vi "convert_image_to_U16.vi"(7 "File Path":path, 8 "error in (no error)":errorcluster, 9 "Image Name":string="untitled", 10 "Convert to U16?":bool, 11 "Image":T1) -> (0 "error out":errorcluster, 2 "unsigned 16bit integer":u16[][](array[numeric]), 3 "Image Out":T1)   [LabVIEW 2013, in "Hamamatsu_C9100-13.lvclass"]
uses:
  Hamamatsu_C9100-13/Hamamatsu_C9100-13.lvclass
  <vilib>/vision/Image Controls.llb/IMAQ Image.ctl
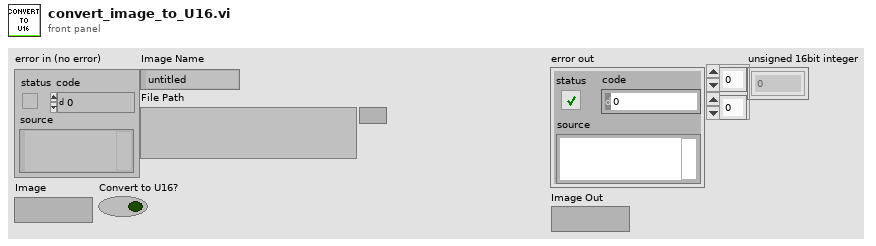
[diagram p1: front panel]
types:
  T1 = typedef "IMAQ Image.ctl" = refnum<image>
  T2 = typedef "Image Type" = u32
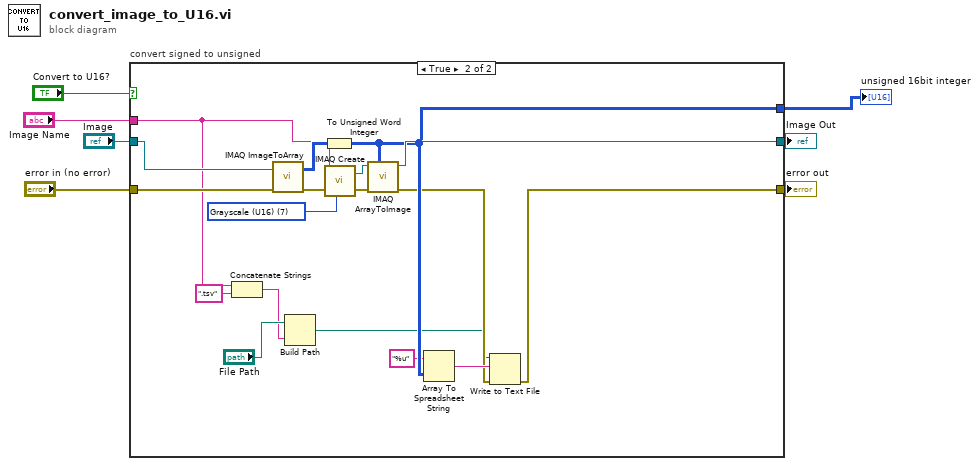
[diagram p0: block diagram]
diagram:
  n1 = case "convert signed to unsigned" shown="True" "Convert to U16?" {
    tunnel: "Image" -> [w9 w20]
    tunnel: [w9 w25] -> w4
    tunnel: "error in (no error)" -> [w8 w21]
    tunnel: [w8 w15] -> w6
    tunnel: "Image Name" -> [_ w12]
    tunnel: [_ w19] -> w1
    frame False {
    }
    frame True {
      w22 = T2 7 items=["Grayscale (U8)", "Grayscale (I16)", "Grayscale (SGL)", "Complex (CSG)", "RGB (U32)", "HSL (U32)", "RGB (U64)", "Grayscale (U16)"] ("Image Type")
      n2 = Concatenate Strings(w12, ".tsv" ("string")) -> (w11:string)
      n3 = call "IMAQ ImageToArray"("error in (no error)"=w21, "Image"=w20) -> ("error out"=w24:errorcluster, "Image Pixels (I16)"=w27:i16[][])  [unwired: 2 in, 3 out]
      n4 = Build Path(base path="File Path", name or relative path=w11) -> (appended path=w13:path)
      n5 = To Unsigned Word Integer(number=w27) -> (unsigned 16bit integer=w19:u16[][])
      n6 = call "IMAQ Create"("Image Name"=w12, "Image Type"=w22, "error in (no error)"=w24) -> ("New Image"=w26:T1, "error out"=w23:errorcluster)  [unwired: 2 in]
      n7 = call "IMAQ ArrayToImage"("Image Pixels (U16)"=w19, "error in (no error)"=w23, "Image"=w26) -> ("error out"=w16:errorcluster, "Image Out"=w25:T1)  [unwired: 7 in]
      n8 = Array To Spreadsheet String(array=w19, 3:"%u" ("format string")) -> (spreadsheet string=w18:string)  [unwired: 1 in]
      n9 = Write to Text File(file (use dialog)=w13, text=w18, error in=w16) -> (error out=w15:errorcluster)  [unwired: 1 in, 2 out]
    }
  }
  "error out" <- w6
  "Image Out" <- w4
  "unsigned 16bit integer" <- w1
